vi "新增产品信息到表格.vi"(11 "新增零件信息":T1) -> (3 "数组":string[](array[string]))   [LabVIEW 2014]
uses:
  ModelInfo.ctl
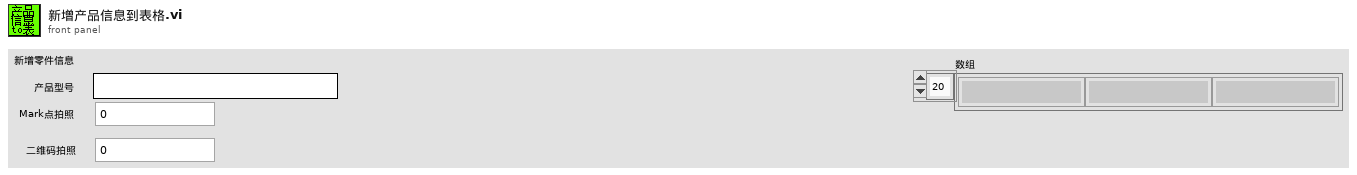
[diagram p1: front panel]
types:
  T1 = typedef "ModelInfo.ctl" = cluster{"产品型号":string, "二维码拍照":u32, "Mark点拍照":u32}
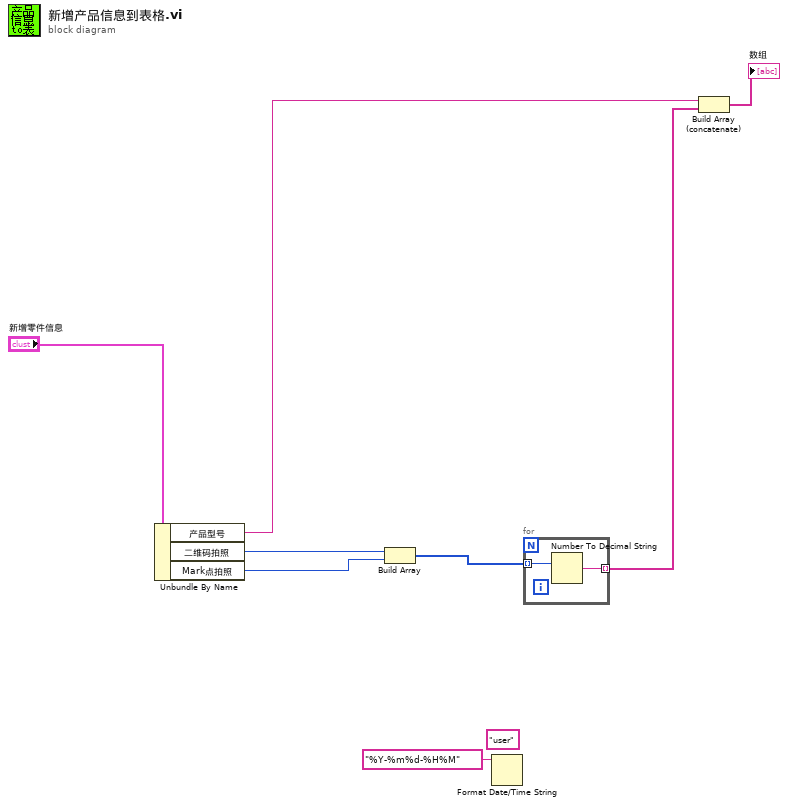
[diagram p0: block diagram]
diagram:
  (unwired) "user" ("元素")
  n1 = Unbundle By Name("新增零件信息") -> ("产品型号"=w1:string, "二维码拍照"=w5:u32, "Mark点拍照"=w4:u32)
  n2 = Build Array(w5, w4) -> (w3:u32[])
  n3 = Format Date/Time String(time format string (%c)="%Y-%m%d-%H%M") -> ()  [unwired: 2 in, 1 out]
  n4 = for {
    tunnel: [w10] -> w2 mode=indexing
    tunnel: w3 -> [w9] mode=indexing
    n5 = Number To Decimal String(number=w9) -> (decimal integer string=w10:string)  [unwired: 1 in]
  }
  n6 = Build Array (concatenate)(w1, w2) -> (→"数组":string[])
